vi "Resize Buffer.vi"(8 "error in (no error)":errorcluster, 11 "Waveform Buffer in":refnum<class "Waveform Buffer.lvclass">) -> (0 "error out":errorcluster, 3 "Waveform Buffer out":refnum<class "Waveform Buffer.lvclass">)   [LabVIEW 2015, in "Waveform Data Logger Engine.lvlib" / "Waveform Buffer.lvclass"]
uses:
  Waveform Buffer.lvclass
  Waveform Buffer.lvclass/Waveform Buffer.ctl
  DBL Waveform Buffer/DBL Waveform Buffer.lvclass
  DBL Waveform Buffer/DBL Waveform Buffer.lvclass/DBL Waveform Buffer.ctl
  CDB Waveform Buffer/CDB Waveform Buffer.lvclass
  Get Buffer Length.vi
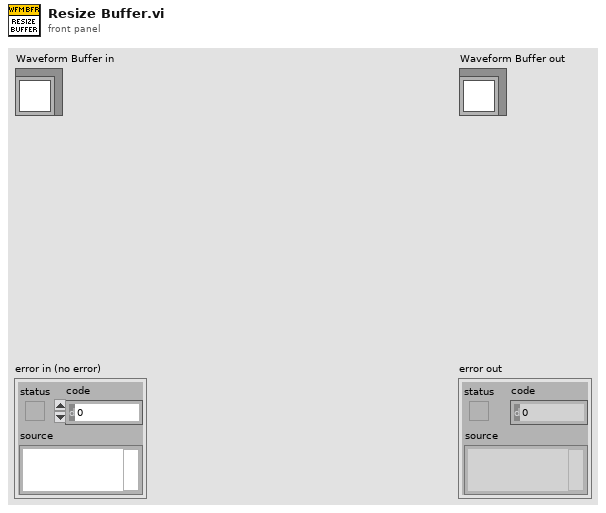
[diagram p1: front panel]
types:
  T1 = typedef "Waveform Data Logger Engine.lvlib/Waveform Buffer.lvclass/Buffer Data Type.ctl" = enum16{"Double", "ComplexDouble"}
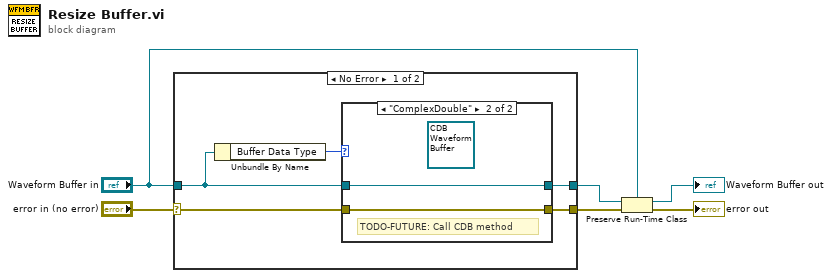
[diagram p0: block diagram]
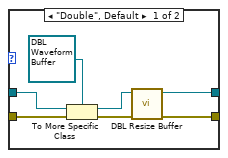
[diagram p2: hidden frame]
diagram:
  n1 = case shown="No Error" "error in (no error)" {
    selector: "error in (no error)" -> [w11 w22]
    tunnel: [w9 w22] -> w3
    tunnel: [w10 w21] -> w5
    tunnel: "Waveform Buffer in" -> [w7 w21]
    frame No Error {
      n2 = Unbundle By Name(w7) -> ("Buffer Data Type"=w8:T1)
      n3 = case shown="\"ComplexDouble\"" w8 {
        tunnel: w7 -> [w13 w19]
        tunnel: w11 -> [w17 w20]
        tunnel: [w18 w20] -> w9
        tunnel: [w12 w19] -> w10
        frame "Double", Default {
          n4 = To More Specific Class(target class=refnum<class "DBL Waveform Buffer.lvclass"> refnum ("Waveform Data Logger Engine.lvlib:DBL Waveform Buffer.lvclass"), reference=w13, error in=w17) -> (specific class reference=w15:refnum<class "DBL Waveform Buffer.lvclass">, error out=w14:errorcluster)
          n5 = call "DBL Resize Buffer.vi"("error in (no error)"=w14, "DBL Waveform Buffer in"=w15) -> ("error out"=w18:errorcluster, "DBL Waveform Buffer out"=w12:refnum<class "DBL Waveform Buffer.lvclass">)  [unwired: 8 in]
        }
        frame "ComplexDouble" {
          (unwired) refnum<class "CDB Waveform Buffer.lvclass"> refnum ("Waveform Data Logger Engine.lvlib:CDB Waveform Buffer.lvclass")
          # "TODO-FUTURE: Call CDB method"
        }
      }
    }
    frame Error {
    }
  }
  n6 = Preserve Run-Time Class(object in=w5, error in=w3, 2:"Waveform Buffer in") -> (object out=→"Waveform Buffer out":refnum<class "Waveform Buffer.lvclass">, error out=→"error out":errorcluster)
